vi "Config Odometry.vi"(8 "error in (no error)":errorcluster, 9 "Ticks per Unit":sgl format="%#_8f", 10 "Wheel Width":sgl format="%#_8f", 11 "Rover in":refnum<class "Rover.lvclass">) -> (0 "error out":errorcluster, 3 "Rover out":refnum<class "Rover.lvclass">)   [LabVIEW 2020, in "Rover.lvlib" / "Rover.lvclass"]
uses:
  Rover.lvclass
  I2C Register.ctl
  Rover.lvclass/Rover.ctl
  <vilib>/MakerHub/LINX/Private/Local IO/LinxI2cWrite.vi
  <vilib>/MakerHub/LINX/Public/Utilities/Check Channel.vi
  <vilib>/MakerHub/LINX/Private/Local IO/Handle Errors.vi
  <vilib>/MakerHub/LINX/Private/Utilties/Generate Error.vi
  <vilib>/MakerHub/LINX/LMH-LINX.lvlib
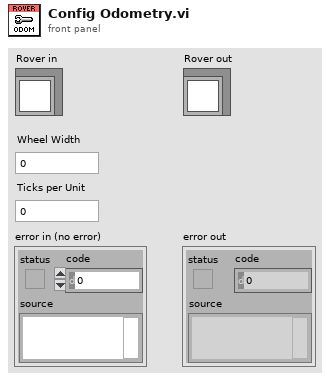
[diagram p1: front panel]
types:
  T1 = typedef "Rover.lvlib/Rover.lvclass/I2C Register.ctl" = enum8{"encA", "encB", "ticksPerUnit", "width", "flags", "velP", "velI", "velD", "velMin", "velMax", "poseX", "poseY", "poseA", "cmdDrive", "cmdTurn", "velocity", "turn", "velL", "velR", "run", "outL", "outR", "outDeadband"}
  T2 = typedef "LMH-LINX.lvlib/LINX Ref.ctl" = cluster{"IO":T3, "Interface":T4, "LINX Device Config":T5}
  T3 = typedef "LMH-LINX.lvlib/Platform.ctl" = enum16{"Remote", "Local"}
  T4 = typedef "LMH-LINX.lvlib/Interface.ctl" = enum16{"Serial", "TCP"}
  T5 = typedef "LMH-LINX.lvlib/Device.lvlib/LINX Device Config.ctl" = cluster{"Interface":T4, "COM Port":refnum<visa-resource-name>, "TCP Configuration":T6, "Device Family":u8, "Device ID":u8, "Device Name":string, "TCP Ref":refnum<k5>, "Channels":T7}
  T6 = typedef "LMH-LINX.lvlib/Device.lvlib/TCP Config.ctl" = cluster{"IP Address":string, "Port":u16}
  T7 = typedef "LMH-LINX.lvlib/Channels.ctl" = cluster{"DI":u8[], "DO":u8[], "AI":u8[], "AO":u8[], "PWM":u8[], "QE":u8[], "UART":u8[], "I2C 2":u8[], "SPI":u8[], "CAN":u8[], "Servo":u8[], "AI Ref (V)":dbl, "AI Resolution (Bits)":u8, "AO Ref (V)":dbl, "AO Resolution (Bits)":u8}
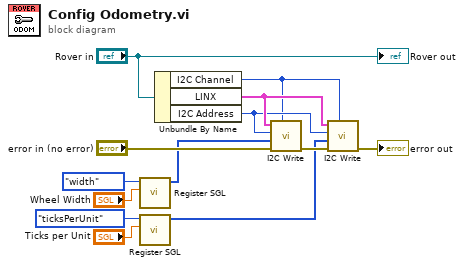
[diagram p0: block diagram]
diagram:
  n1 = call "Register SGL.vi"("Value"="Wheel Width", "Register"=I2C_Register."width") -> ("Data"=w2:u8[])  [unwired: 9 in]
  n2 = call "Register SGL.vi"("Value"="Ticks per Unit", "Register"=I2C_Register."ticksPerUnit") -> ("Data"=w1:u8[])  [unwired: 9 in]
  n3 = Unbundle By Name("Rover in") -> ("I2C Channel"=w5:u8, "LINX"=w7:T2, "I2C Address"=w6:u8)
  n4 = call <vilib>:"I2C Write.vi"("I2C Channel"=w5, "Error In"="error in (no error)", "Data"=w2, "I2C Slave Address (0)"=w6, "LINX Resource"=w7) -> ("Error Out"=w4:errorcluster)  [unwired: 5 in, 1 out]
  n5 = call <vilib>:"I2C Write.vi"("I2C Channel"=w5, "Error In"=w4, "Data"=w1, "I2C Slave Address (0)"=w6, "LINX Resource"=w7) -> ("Error Out"=→"error out":errorcluster)  [unwired: 5 in, 1 out]
  "Rover out" <- "Rover in"
